vi "LV Exp1.vi"() -> ()   [LabVIEW 2009]
uses:
  <vilib>/NXT/Block Support/NXT_InputPort.ctl
  <vilib>/NXT/Dual Mode Library/Display/drawText.vi
panel:
  in  "stop":bool
  out "LED":bool
  out "Switch Status":string
  # "HiTechnic Experimenter's Kit\n\n                        Experiment 1 - Introduction\nThis program reads the status of the switch on A0 and\nif the switch is closed (pressed), the LED on B0 is truned on.\n\nSee Experimenter's Kit Handbook for the SuperPro for\nmore information or go to www.hitechnic.com.\n\n(c) HiTechnic 2011"
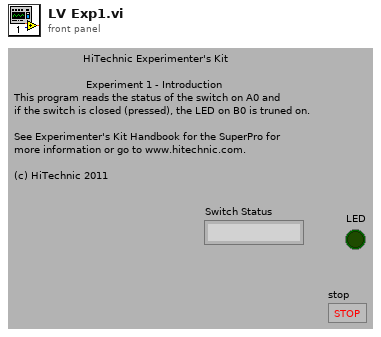
[diagram p1: front panel]
types:
  T1 = typedef "NXT_InputPort.ctl" = u8
  T2 = typedef "LVHSConnector.ctl" = cluster{"error":errorcluster, "address":string, "NXT #":i32, "Show Error":bool, "Connection":u16}
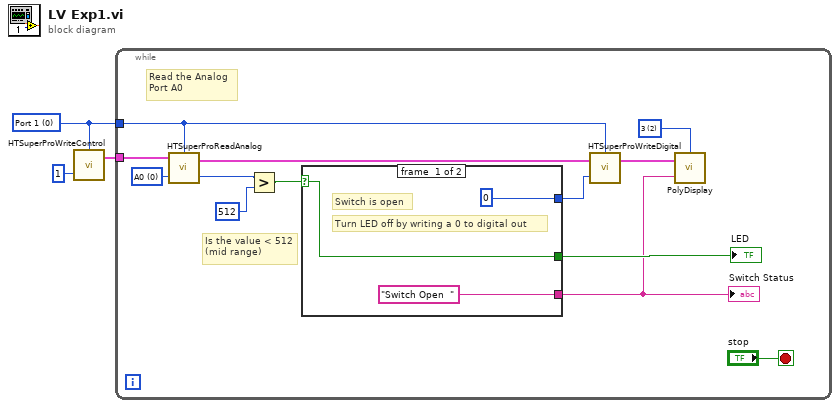
[diagram p0: block diagram]
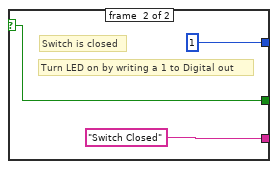
[diagram p2: hidden frame]
diagram:
  w1 = T1 0 items=["Port 1", "Port 2", "Port 3", "Port 4"] ("Port")
  n1 = call "HTSuperProWriteControl.vi"("Digital Value"=u8 1, "Port"=w1) -> ("NXT"=w3:T2)  [unwired: 3 in]
  n2 = while {
    tunnel: w1 -> [w13]
    tunnel: w3 -> [w16]
    stop <- "stop" stop-if-true
    w4 = u8 0 items=["A0", "A1", "A2", "A3"] ("Analog Port")
    w6 = i16 2 items=["1", "2", "3", "4", "5", "6", "7", "8"] ("Line")
    # "Is the value < 512\n(mid range)"
    # "Read the Analog\nPort A0"
    n3 = call "HTSuperProReadAnalog.vi"("Analog Port"=w4, "NXT"=w16, "Port"=w13) -> ("Analog Value"=w9:i16, "NXT"=w15:T2)  [unwired: 1 in]
    n4 = Greater?(x=w9, y=i16 512) -> (0:w10:bool)
    n5 = case shown="True" w10 {
      selector: w10 -> [w17 w20]
      tunnel: ["Switch Open  " "Switch Closed"] -> w5
      tunnel: [u8 0 ("Digital Value") u8 1 ("Digital Value")] -> w14
      tunnel: [w17 w20] -> w12
      frame #0 {
        # "Turn LED off by writing a 0 to digital out"
        # "Switch is open"
      }
      frame #1 {
        # "Turn LED on by writing a 1 to Digital out"
        # "Switch is closed"
      }
    }
    "LED" <- w12
    "Switch Status" <- w5
    n6 = call "HTSuperProWriteDigital.vi"("Digital Value"=w14, "NXT"=w15, "Port"=w13) -> ("NXT"=w7:T2)  [unwired: 2 in]
    n7 = call-poly <vilib>:"PolyDisplay.vi"("Text"=w5, "NXT"=w7, "Line"=w6) -> ()  [unwired: 1 in, 1 out]
  }
